vi "VI Tree.vi"   [LabVIEW 2016, in "Keithley 6517.lvlib"]
doc: "This is the instrument driver for Keithley 6517 A/B and 6514. The VI Tree displays all the user-callable VIs of the instrument driver in an organized table."
uses:
  <instrlib>/Keithley 6517/Keithley 6517.lvlib
panel:
  # "(c) 2016-2017 National Instruments.  ALL RIGHTS RESERVED."
  # "SEE DIAGRAM\nFOR VI TREE."
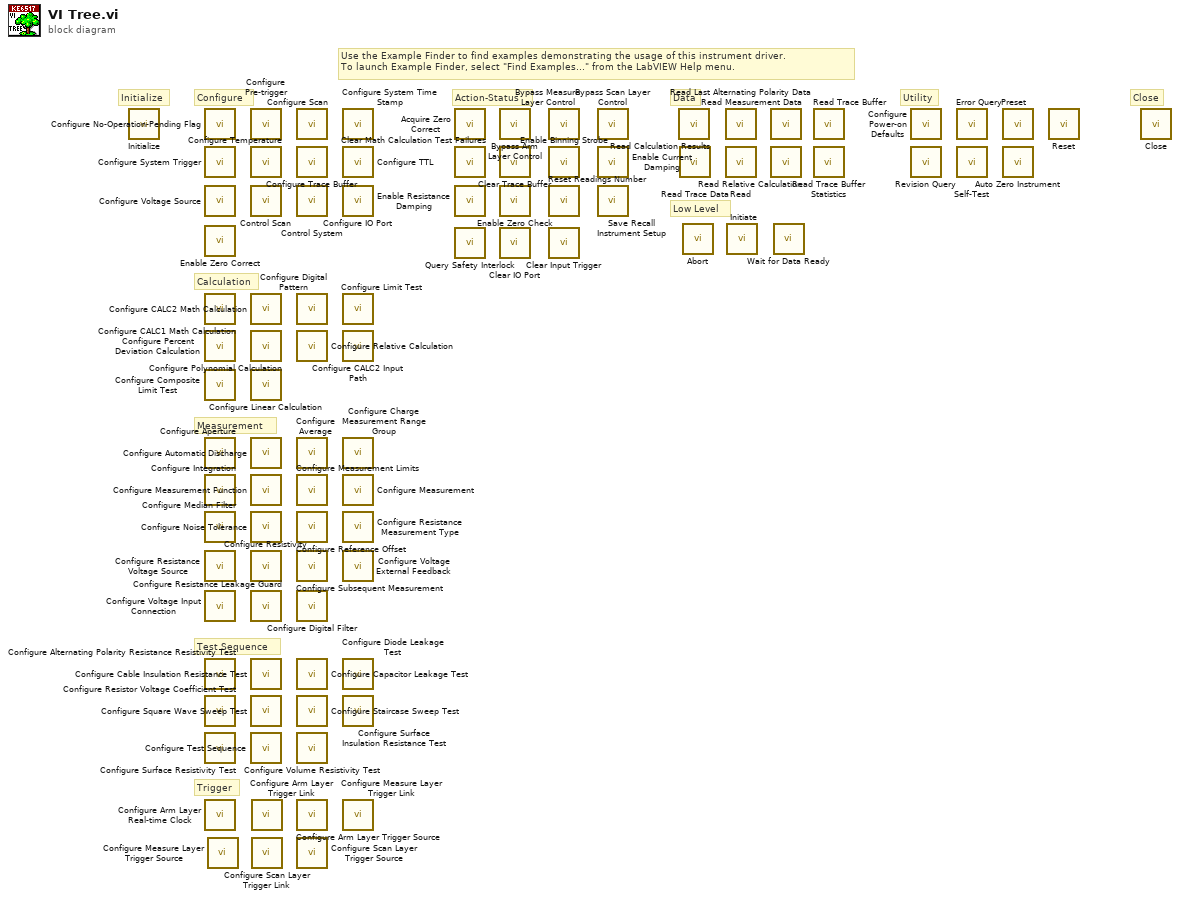
[diagram p0: block diagram]
diagram:
  # "Low Level"
  # "Close"
  # "Utility"
  # "Data"
  # "Trigger"
  # "Test Sequence"
  # "Measurement"
  # "Calculation"
  # "Configure"
  # "Action-Status"
  # "Initialize"
  # "Use the Example Finder to find examples demonstrating the usage of this instrument driver.\nTo launch Example Finder, select \"Find Examples...\" from the LabVIEW Help menu."
  n1 = call <instrlib>:"Initialize.vi"() -> ()  [unwired: 10 in, 2 out]
  n2 = call <instrlib>:"Configure No-Operation-Pending Flag.vi"() -> ()  [unwired: 10 in, 2 out]
  n3 = call <instrlib>:"Configure System Trigger.vi"() -> ()  [unwired: 10 in, 2 out]
  n4 = call <instrlib>:"Configure Voltage Source.vi"() -> ()  [unwired: 14 in, 2 out]
  n5 = call <instrlib>:"Enable Zero Correct.vi"() -> ()  [unwired: 10 in, 2 out]
  n6 = call <instrlib>:"Configure CALC1 Math Calculation.vi"() -> ()  [unwired: 10 in, 2 out]
  n7 = call <instrlib>:"Configure Percent Deviation Calculation.vi"() -> ()  [unwired: 10 in, 2 out]
  n8 = call <instrlib>:"Configure Composite Limit Test.vi"() -> ()  [unwired: 10 in, 2 out]
  n9 = call <instrlib>:"Configure Aperture.vi"() -> ()  [unwired: 10 in, 2 out]
  n10 = call <instrlib>:"Configure Integration.vi"() -> ()  [unwired: 10 in, 2 out]
  n11 = call <instrlib>:"Configure Median Filter.vi"() -> ()  [unwired: 10 in, 2 out]
  n12 = call <instrlib>:"Configure Resistance Voltage Source.vi"() -> ()  [unwired: 14 in, 2 out]
  n13 = call <instrlib>:"Configure Voltage Input Connection.vi"() -> ()  [unwired: 10 in, 2 out]
  n14 = call <instrlib>:"Configure Alternating Polarity Resistance Resistivity Test.vi"() -> ()  [unwired: 10 in, 2 out]
  n15 = call <instrlib>:"Configure Resistor Voltage Coefficient Test.vi"() -> ()  [unwired: 10 in, 2 out]
  n16 = call <instrlib>:"Configure Surface Resistivity Test.vi"() -> ()  [unwired: 14 in, 2 out]
  n17 = call <instrlib>:"Configure Arm Layer Real-time Clock.vi"() -> ()  [unwired: 14 in, 2 out]
  n18 = call <instrlib>:"Configure Measure Layer Trigger Source.vi"() -> ()  [unwired: 10 in, 2 out]
  n19 = call <instrlib>:"Configure Pre-trigger.vi"() -> ()  [unwired: 10 in, 2 out]
  n20 = call <instrlib>:"Configure Temperature.vi"() -> ()  [unwired: 10 in, 2 out]
  n21 = call <instrlib>:"Control Scan.vi"() -> ()  [unwired: 10 in, 2 out]
  n22 = call <instrlib>:"Configure CALC2 Math Calculation.vi"() -> ()  [unwired: 10 in, 2 out]
  n23 = call <instrlib>:"Configure Polynomial Calculation.vi"() -> ()  [unwired: 10 in, 2 out]
  n24 = call <instrlib>:"Configure Linear Calculation.vi"() -> ()  [unwired: 10 in, 2 out]
  n25 = call <instrlib>:"Configure Automatic Discharge.vi"() -> ()  [unwired: 10 in, 2 out]
  n26 = call <instrlib>:"Configure Measurement Function.vi"() -> ()  [unwired: 10 in, 2 out]
  n27 = call <instrlib>:"Configure Noise Tolerance.vi"() -> ()  [unwired: 10 in, 2 out]
  n28 = call <instrlib>:"Configure Resistivity.vi"() -> ()  [unwired: 10 in, 2 out]
  n29 = call <instrlib>:"Configure Resistance Leakage Guard.vi"() -> ()  [unwired: 10 in, 2 out]
  n30 = call <instrlib>:"Configure Cable Insulation Resistance Test.vi"() -> ()  [unwired: 10 in, 2 out]
  n31 = call <instrlib>:"Configure Square Wave Sweep Test.vi"() -> ()  [unwired: 10 in, 2 out]
  n32 = call <instrlib>:"Configure Test Sequence.vi"() -> ()  [unwired: 10 in, 2 out]
  n33 = call <instrlib>:"Configure Arm Layer Trigger Link.vi"() -> ()  [unwired: 10 in, 2 out]
  n34 = call <instrlib>:"Configure Scan Layer Trigger Link.vi"() -> ()  [unwired: 10 in, 2 out]
  n35 = call <instrlib>:"Configure Scan.vi"() -> ()  [unwired: 14 in, 2 out]
  n36 = call <instrlib>:"Configure Trace Buffer.vi"() -> ()  [unwired: 10 in, 2 out]
  n37 = call <instrlib>:"Control System.vi"() -> ()  [unwired: 14 in, 2 out]
  n38 = call <instrlib>:"Configure Digital Pattern.vi"() -> ()  [unwired: 10 in, 2 out]
  n39 = call <instrlib>:"Configure Relative Calculation.vi"() -> ()  [unwired: 14 in, 2 out]
  n40 = call <instrlib>:"Configure Average.vi"() -> ()  [unwired: 10 in, 2 out]
  n41 = call <instrlib>:"Configure Measurement Limits.vi"() -> ()  [unwired: 10 in, 2 out]
  n42 = call <instrlib>:"Configure Reference Offset.vi"() -> ()  [unwired: 10 in, 2 out]
  n43 = call <instrlib>:"Configure Subsequent Measurement.vi"() -> ()  [unwired: 10 in, 2 out]
  n44 = call <instrlib>:"Configure Digital Filter.vi"() -> ()  [unwired: 14 in, 2 out]
  n45 = call <instrlib>:"Configure Capacitor Leakage Test.vi"() -> ()  [unwired: 10 in, 2 out]
  n46 = call <instrlib>:"Configure Staircase Sweep Test.vi"() -> ()  [unwired: 10 in, 2 out]
  n47 = call <instrlib>:"Configure Volume Resistivity Test.vi"() -> ()  [unwired: 14 in, 2 out]
  n48 = call <instrlib>:"Configure Arm Layer Trigger Source.vi"() -> ()  [unwired: 10 in, 2 out]
  n49 = call <instrlib>:"Configure Scan Layer Trigger Source.vi"() -> ()  [unwired: 10 in, 2 out]
  n50 = call <instrlib>:"Configure System Time Stamp.vi"() -> ()  [unwired: 10 in, 2 out]
  n51 = call <instrlib>:"Configure TTL.vi"() -> ()  [unwired: 14 in, 2 out]
  n52 = call <instrlib>:"Configure IO Port.vi"() -> ()  [unwired: 14 in, 2 out]
  n53 = call <instrlib>:"Configure Limit Test.vi"() -> ()  [unwired: 14 in, 2 out]
  n54 = call <instrlib>:"Configure CALC2 Input Path.vi"() -> ()  [unwired: 10 in, 2 out]
  n55 = call <instrlib>:"Configure Charge Measurement Range Group.vi"() -> ()  [unwired: 10 in, 2 out]
  n56 = call <instrlib>:"Configure Measurement.vi"() -> ()  [unwired: 10 in, 2 out]
  n57 = call <instrlib>:"Configure Resistance Measurement Type.vi"() -> ()  [unwired: 10 in, 2 out]
  n58 = call <instrlib>:"Configure Voltage External Feedback.vi"() -> ()  [unwired: 10 in, 2 out]
  n59 = call <instrlib>:"Configure Diode Leakage Test.vi"() -> ()  [unwired: 10 in, 2 out]
  n60 = call <instrlib>:"Configure Surface Insulation Resistance Test.vi"() -> ()  [unwired: 10 in, 2 out]
  n61 = call <instrlib>:"Configure Measure Layer Trigger Link.vi"() -> ()  [unwired: 10 in, 2 out]
  n62 = call <instrlib>:"Acquire Zero Correct.vi"() -> ()  [unwired: 10 in, 2 out]
  n63 = call <instrlib>:"Clear Math Calculation Test Failures .vi"() -> ()  [unwired: 10 in, 2 out]
  n64 = call <instrlib>:"Enable Resistance Damping.vi"() -> ()  [unwired: 10 in, 2 out]
  n65 = call <instrlib>:"Query Safety Interlock.vi"() -> ()  [unwired: 9 in, 3 out]
  n66 = call <instrlib>:"Bypass Arm Layer Control.vi"() -> ()  [unwired: 10 in, 2 out]
  n67 = call <instrlib>:"Clear Trace Buffer.vi"() -> ()  [unwired: 10 in, 2 out]
  n68 = call <instrlib>:"Enable Zero Check.vi"() -> ()  [unwired: 10 in, 2 out]
  n69 = call <instrlib>:"Clear IO Port.vi"() -> ()  [unwired: 10 in, 2 out]
  n70 = call <instrlib>:"Bypass Measure Layer Control.vi"() -> ()  [unwired: 10 in, 2 out]
  n71 = call <instrlib>:"Enable Binning Strobe.vi"() -> ()  [unwired: 10 in, 2 out]
  n72 = call <instrlib>:"Reset Readings Number.vi"() -> ()  [unwired: 10 in, 2 out]
  n73 = call <instrlib>:"Clear Input Trigger.vi"() -> ()  [unwired: 10 in, 2 out]
  n74 = call <instrlib>:"Bypass Scan Layer Control.vi"() -> ()  [unwired: 10 in, 2 out]
  n75 = call <instrlib>:"Enable Current Damping.vi"() -> ()  [unwired: 10 in, 2 out]
  n76 = call <instrlib>:"Save Recall Instrument Setup.vi"() -> ()  [unwired: 10 in, 2 out]
  n77 = call <instrlib>:"Read Calculation Results.vi"() -> ()  [unwired: 9 in, 7 out]
  n78 = call <instrlib>:"Read Trace Data.vi"() -> ()  [unwired: 9 in, 3 out]
  n79 = call <instrlib>:"Abort.vi"() -> ()  [unwired: 10 in, 2 out]
  n80 = call <instrlib>:"Read Last Alternating Polarity Data.vi"() -> ()  [unwired: 9 in, 3 out]
  n81 = call <instrlib>:"Read.vi"() -> ()  [unwired: 9 in, 3 out]
  n82 = call <instrlib>:"Initiate.vi"() -> ()  [unwired: 10 in, 2 out]
  n83 = call <instrlib>:"Read Measurement Data.vi"() -> ()  [unwired: 9 in, 3 out]
  n84 = call <instrlib>:"Read Relative Calculation.vi"() -> ()  [unwired: 9 in, 3 out]
  n85 = call <instrlib>:"Wait for Data Ready.vi"() -> ()  [unwired: 10 in, 2 out]
  n86 = call <instrlib>:"Read Trace Buffer.vi"() -> ()  [unwired: 7 in, 5 out]
  n87 = call <instrlib>:"Read Trace Buffer Statistics.vi"() -> ()  [unwired: 9 in, 7 out]
  n88 = call <instrlib>:"Configure Power-on Defaults.vi"() -> ()  [unwired: 10 in, 2 out]
  n89 = call <instrlib>:"Revision Query.vi"() -> ()  [unwired: 8 in, 4 out]
  n90 = call <instrlib>:"Error Query.vi"() -> ()  [unwired: 8 in, 4 out]
  n91 = call <instrlib>:"Self-Test.vi"() -> ()  [unwired: 8 in, 4 out]
  n92 = call <instrlib>:"Preset.vi"() -> ()  [unwired: 10 in, 2 out]
  n93 = call <instrlib>:"Auto Zero Instrument.vi"() -> ()  [unwired: 10 in, 2 out]
  n94 = call <instrlib>:"Reset.vi"() -> ()  [unwired: 10 in, 2 out]
  n95 = call <instrlib>:"Close.vi"() -> ()  [unwired: 11 in, 1 out]
